vi "5492_GlobalShooting.vi"() -> ()   [LabVIEW 2016]
panel:
  out "Shooting":bool
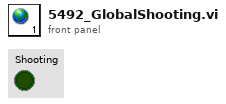
[diagram p1: front panel]
diagram:
